vi "Backprop.vi"(0 "Target":dbl, 5 "Training Constant":dbl, 7 "Function Final Layer":u16, 9 "Output":dbl, 11 "Hidden Outputs":dbl[](array[numeric]), 12 "Function Hidden Layer":u16, 13 "Inputs":dbl[](array[numeric]), 14 "Hidden Weights":dbl[][](array[numeric]), 15 "Final Weights":dbl[](array[numeric])) -> (4 "Hidden Error":dbl[](array[numeric]), 6 "Final Error for Back Prop":dbl, 8 "New Output Weights":dbl[](array[numeric]), 10 "New Hidden Weights":dbl[][](array[numeric]))   [LabVIEW 2009]
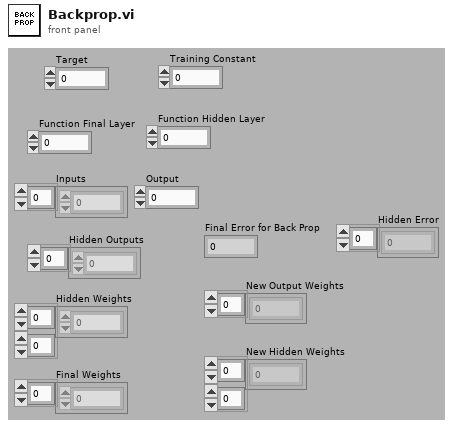
[diagram p1: front panel]
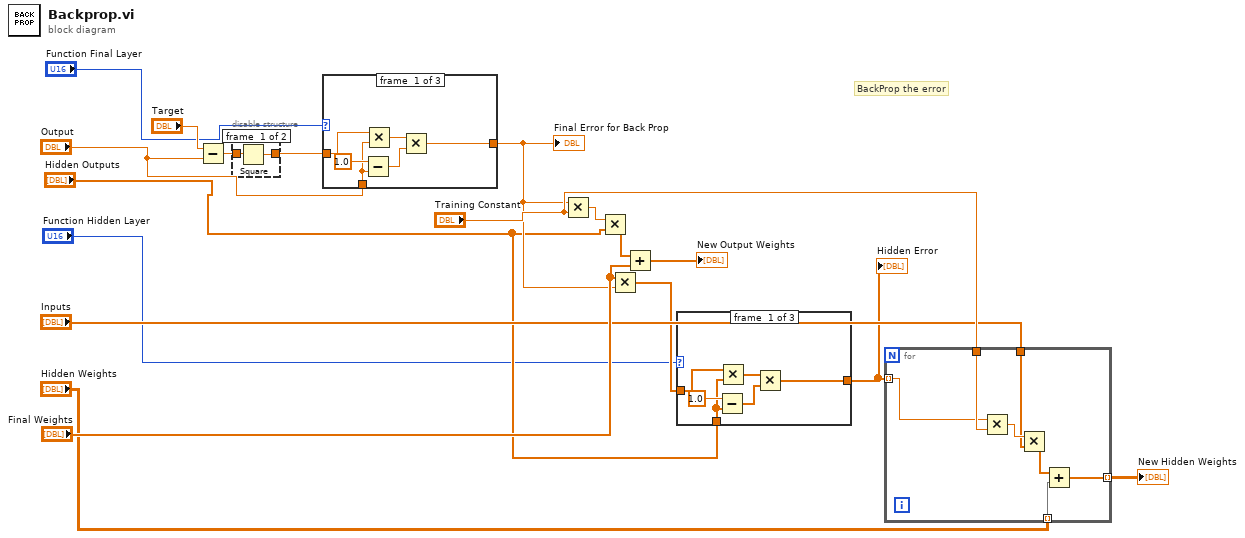
[diagram p0: block diagram]
diagram:
  # "BackProp the error"
  n1 = Subtract(x="Target", y="Output") -> (x-y=w9:dbl)
  n2 = disable-structure shown="Enabled" {
    disable-tunnel: w9 -> [w20 w21]
    disable-tunnel: [w19 w21] -> w6
    frame #0 {
      n3 = Square(x=w20) -> (x^2=w19:dbl)
    }
    frame #1 {
    }
  }
  n4 = case shown="0, Default" "Function Final Layer" {
    tunnel: w6 -> [w23 w28 w29]
    tunnel: "Output" -> [w24 _ _]
    tunnel: [w22 w28 w29] -> w14
    frame #0 {
      n5 = Subtract(x=1.0, y=w24) -> (x-y=w26:dbl)
      n6 = Multiply(x=w23, y=w24) -> (x*y=w27:dbl)
      n7 = Multiply(x=w27, y=w26) -> (x*y=w22:dbl)
    }
    frame #1 {
    }
    frame #2 {
    }
  }
  "Final Error for Back Prop" <- w14
  n8 = Multiply(x=w14, y="Training Constant") -> (x*y=w11:dbl)
  n9 = Multiply(x=w11, y="Hidden Outputs") -> (x*y=w12:dbl[])
  n10 = Multiply(x="Final Weights", y=w14) -> (x*y=w4:dbl[])
  n11 = Add(x=w12, y="Final Weights") -> (x+y=→"New Output Weights":dbl[])
  n12 = case shown="0, Default" "Function Hidden Layer" {
    tunnel: w4 -> [w32 w36 w37]
    tunnel: "Hidden Outputs" -> [w30 _ _]
    tunnel: [w31 w36 w37] -> w2
    frame #0 {
      n13 = Subtract(x=1.0, y=w30) -> (x-y=w34:dbl[])
      n14 = Multiply(x=w32, y=w30) -> (x*y=w35:dbl[])
      n15 = Multiply(x=w35, y=w34) -> (x*y=w31:dbl[])
    }
    frame #1 {
    }
    frame #2 {
    }
  }
  "Hidden Error" <- w2
  n16 = for {
    tunnel: w2 -> [w38] mode=indexing
    tunnel: "Training Constant" -> [w42]
    tunnel: "Hidden Weights" -> [w41] mode=indexing
    tunnel: "Inputs" -> [w40]
    tunnel: [w39] -> w17 mode=indexing
    n17 = Multiply(x=w38, y=w42) -> (x*y=w43:dbl)
    n18 = Multiply(x=w43, y=w40) -> (x*y=w44:dbl[])
    n19 = Add(x=w44, y=w41) -> (x+y=w39:dbl[])
  }
  "New Hidden Weights" <- w17
